vi "TurnToAngle.vi"(10 "Target Angle":dbl=30.0, 11 "Robot Angle":dbl=-0.04000000000000625) -> (1 "Error":dbl=30.04000000000002, 2 "Right Setpoint":dbl=-0.3004000000000002, 3 "Left Setpoint":dbl=0.3004000000000002)   [LabVIEW 2018]
panel:
  in  "Min Output":dbl=0.3
  in  "Max Output":dbl=0.8
  in  "iZone":dbl
  in  "kD":dbl=0.012
  in  "kI":dbl
  in  "kP":dbl=0.01
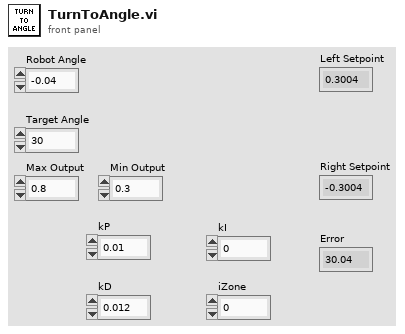
[diagram p1: front panel]
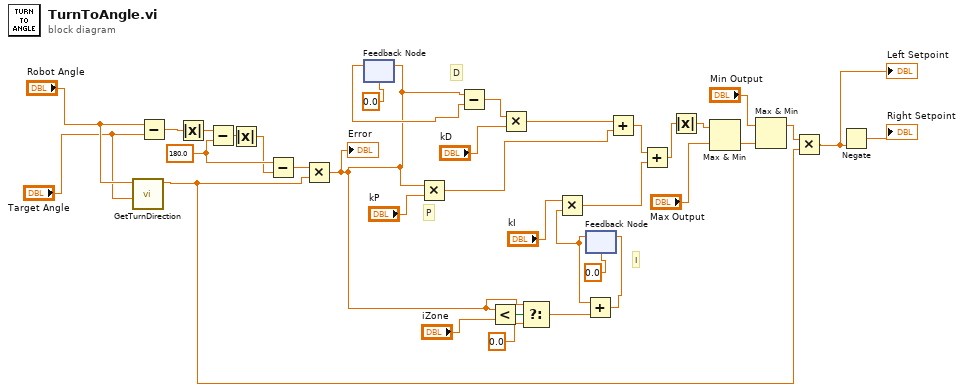
[diagram p0: block diagram]
diagram:
  w32 = 180.0
  # "P"
  # "D"
  # "I"
  n1 = call "GetTurnDirection.vi"("Target Angle"="Target Angle", "Robot Angle"="Robot Angle") -> ("Numeric"=w1:dbl)  [unwired: 9 in]
  n2 = Subtract(x="Robot Angle", y="Target Angle") -> (x-y=w35:dbl)
  n3 = Absolute Value(x=w35) -> (abs(x)=w34:dbl)
  n4 = Subtract(x=w34, y=w32) -> (x-y=w33:dbl)
  n5 = Absolute Value(x=w33) -> (abs(x)=w31:dbl)
  n6 = Subtract(x=w32, y=w31) -> (x-y=w9:dbl)
  n7 = Multiply(x=w9, y=w1) -> (x*y=w8:dbl)
  "Error" <- w8
  n8 = feedback-in #1(w8) -> ()
  n9 = feedback #1(0.0) -> (w21:dbl)
  n10 = Multiply(x=w8, y="kP") -> (x*y=w16:dbl)
  n11 = Subtract(x=w8, y=w21) -> (x-y=w19:dbl)
  n12 = Less?(x=w8, y="iZone") -> (x < y?=w28:bool)
  n13 = Multiply(x=w19, y="kD") -> (x*y=w17:dbl)
  n14 = Select(t=w8, s=w28, f=0.0) -> (s? t:f=w24:dbl)
  n15 = feedback #2(0.0) -> (w22:dbl)
  n16 = Multiply(x="kI", y=w22) -> (x*y=w14:dbl)
  n17 = Add(x=w22, y=w24) -> (x+y=w26:dbl)
  n18 = feedback-in #2(w26) -> ()
  n19 = Add(x=w17, y=w16) -> (x+y=w15:dbl)
  n20 = Add(x=w15, y=w14) -> (x+y=w4:dbl)
  n21 = Absolute Value(x=w4) -> (abs(x)=w5:dbl)
  n22 = Max & Min(x=w5, y="Max Output") -> (min(x,y)=w7:dbl)  [unwired: 1 out]
  n23 = Max & Min(x="Min Output", y=w7) -> (max(x,y)=w2:dbl)  [unwired: 1 out]
  n24 = Multiply(x=w2, y=w1) -> (x*y=w3:dbl)
  "Left Setpoint" <- w3
  n25 = Negate(x=w3) -> (-x=→"Right Setpoint":dbl)
